vi "Untitled 1.vi"(7 "Sheet Name":string, 8 "error in":errorcluster, 9 "Value":bool, 10 "Cell Address":string, 11 "SpreadsheetDoc in":refnum<k24>) -> (0 "error out":errorcluster, 3 "SpreadsheetDoc out":refnum<k24>)   [LabVIEW 2021, in "Open Xml.lvlib"]
uses:
  Open Xml.lvlib
  D:/git/Open-Xml-LabVIEW/dll/DocumentFormat.OpenXml.dll
  dll/DocumentFormat.OpenXml.dll
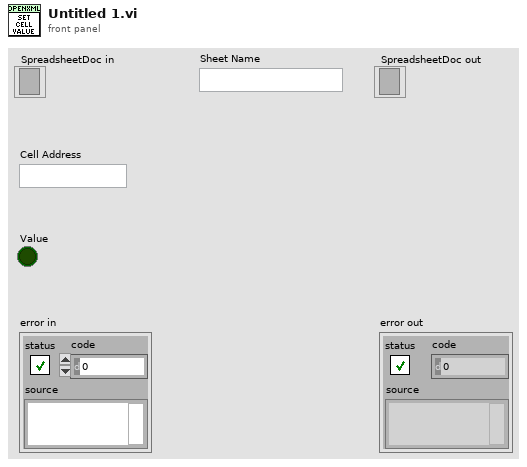
[diagram p1: front panel]
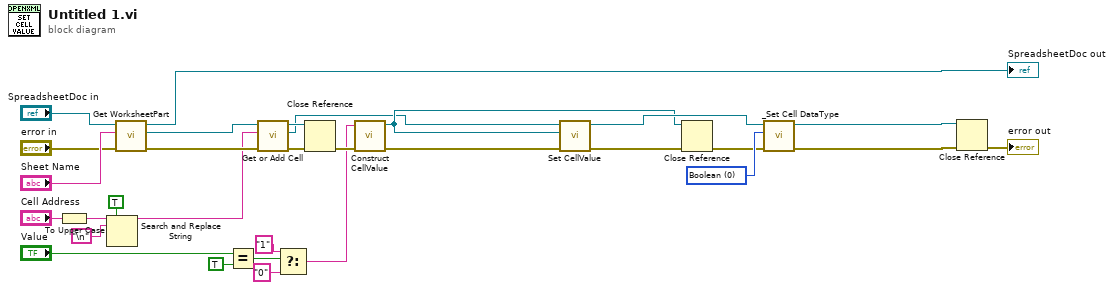
[diagram p0: block diagram]
diagram:
  w11 = 0 items=["Boolean", "Number", "Error", "SharedString", "String", "InlineString", "Date"] ("Datatype")
  n1 = To Upper Case(1:"Cell Address") -> (0:w19:string)
  n2 = Search and Replace String(replace all?=TRUE ("replace all? (F)"), input string=w19, search string="\n") -> (result string=w18:string)  [unwired: 5 in, 3 out]
  n3 = call "Get WorksheetPart.vi"("error in"="error in", "Sheet Name"="Sheet Name", "SpreadsheetDocument in"="SpreadsheetDoc in") -> ("error out"=w26:errorcluster, "WorksheetPart"=w25:refnum<k24>, "SpreadsheetDocument out"=→"SpreadsheetDoc out":refnum<k24>)  [unwired: 6 in]
  n4 = Equal?(x="Value", y=TRUE) -> (x = y?=w3:bool)
  n5 = call "Get or Add Cell.vi"("error in"=w26, "Cell Address"=w18, "Worksheetpart in"=w25) -> ("error out"=w15:errorcluster, "Cell"=w6:refnum<k24>, "WorksheetPart out"=w7:refnum<k24>)  [unwired: 6 in]
  n6 = Select(t="1", s=w3, f="0" ("t")) -> (s? t:f=w2:string)
  n7 = Close Reference(reference=w7, error in (no error)=w15) -> (error out=w8:errorcluster)
  n8 = call "Construct CellValue.vi"("error in"=w8, "Text"=w2) -> ("error out"=w14:errorcluster, "CellValue out"=w9:refnum<k24>)  [unwired: 8 in]
  n9 = call "Set CellValue.vi"("error in"=w14, "CellValue in"=w9, "Cell in"=w6) -> ("error out"=w12:errorcluster, "Cell out"=w13:refnum<k24>)  [unwired: 7 in]
  n10 = Close Reference(reference=w9, error in (no error)=w12) -> (error out=w10:errorcluster)
  n11 = call "_Set Cell DataType.vi"("error in"=w10, "Datatype"=w11, "Cell in"=w13) -> ("error out"=w24:errorcluster, "Cell out"=w23:refnum<k24>)  [unwired: 7 in]
  n12 = Close Reference(reference=w23, error in (no error)=w24) -> (error out=→"error out":errorcluster)
